vi "Cross Product.vi"(9 "Vector 2":cluster{"X":sgl, "Y":sgl, "Z":sgl}, 11 "Vector 1":cluster{"X":sgl, "Y":sgl, "Z":sgl}) -> (3 "Vector Out":cluster{"X":sgl, "Y":sgl, "Z":sgl})   [LabVIEW 2017, in "3D Plot.lvclass"]
uses:
  <vilib>/Math Plots/3D Math Plots/3D Plot/3D Plot/3D Plot.lvclass
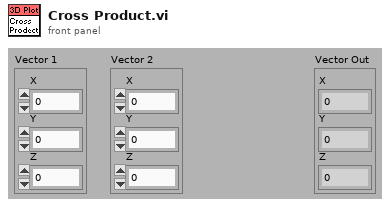
[diagram p1: front panel]
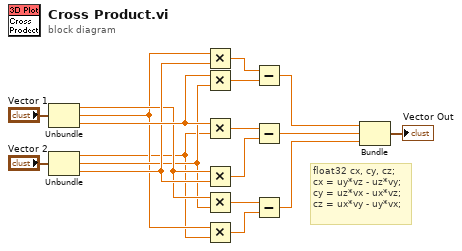
[diagram p0: block diagram]
diagram:
  # "float32 cx, cy, cz;\ncx = uy*vz - uz*vy;\ncy = uz*vx - ux*vz;\ncz = ux*vy - uy*vx;"
  n1 = Unbundle("Vector 1") -> ("X"=w8:sgl, "Y"=w5:sgl, "Z"=w12:sgl)
  n2 = Unbundle("Vector 2") -> ("X"=w4:sgl, "Y"=w7:sgl, "Z"=w11:sgl)
  n3 = Multiply(x=w5, y=w11) -> (x*y=w15:sgl)
  n4 = Multiply(x=w12, y=w7) -> (x*y=w14:sgl)
  n5 = Multiply(x=w12, y=w4) -> (x*y=w10:sgl)
  n6 = Multiply(x=w8, y=w11) -> (x*y=w9:sgl)
  n7 = Multiply(x=w8, y=w7) -> (x*y=w2:sgl)
  n8 = Multiply(x=w5, y=w4) -> (x*y=w3:sgl)
  n9 = Subtract(x=w15, y=w14) -> (x-y=w13:sgl)
  n10 = Subtract(x=w10, y=w9) -> (x-y=w6:sgl)
  n11 = Subtract(x=w2, y=w3) -> (x-y=w1:sgl)
  n12 = Bundle(w13, w6, w1) -> (→"Vector Out":cluster{sgl, sgl, sgl})  [unwired: 1 out]
